vi "Read setpoint.vi"(8 "error in (no error)":errorcluster, 11 "SetSpectTempSetpoint in":refnum<class "setSpectTempSetpoint.lvclass">) -> (0 "error out":errorcluster, 2 "setpoint":sgl, 3 "SetSpectTempSetpoint out":refnum<class "setSpectTempSetpoint.lvclass">)   [LabVIEW 2016, in "Commands.lvlib" / "setSpectTempSetpoint.lvclass"]
uses:
  setSpectTempSetpoint.lvclass
  setSpectTempSetpoint.lvclass/setSpectTempSetpoint.ctl
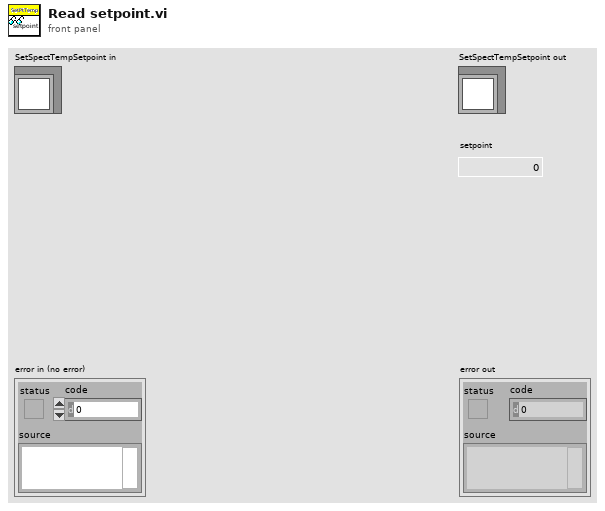
[diagram p1: front panel]
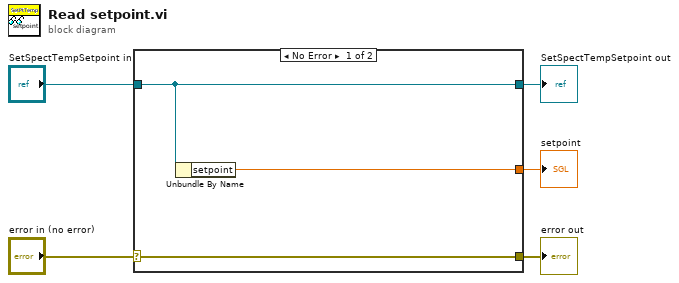
[diagram p0: block diagram]
diagram:
  n1 = case shown="No Error" "error in (no error)" {
    selector: "error in (no error)" -> [w8 w9]
    tunnel: [w8 w9] -> w4
    tunnel: [w7 w10] -> w2
    tunnel: "SetSpectTempSetpoint in" -> [w7 w10]
    tunnel: [w6 _] -> w1
    frame No Error {
      n2 = Unbundle By Name(w7) -> ("setpoint"=w6:sgl)
    }
    frame Error {
    }
  }
  "error out" <- w4
  "SetSpectTempSetpoint out" <- w2
  "setpoint" <- w1
